vi "camera_config.vi"(7 "Cam Delay":dbl=0.5, 8 "error in (no error)":errorcluster, 9 "Sub Region":T1={"Horizontal Offset"=768, "Vertical Offset"=960, "Horizontal Size"=512, "Vertical Size"=128}, 10 "Exposure Time(s)":dbl=0.00199, 11 "Handle in":u32) -> (0 "error out":errorcluster, 3 "Handle out":u32)   [LabVIEW 2017]
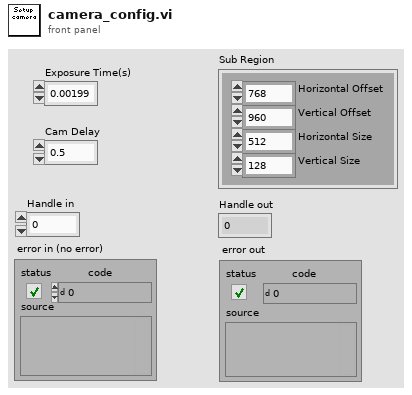
[diagram p1: front panel]
types:
  T1 = cluster{"Horizontal Offset":i32, "Vertical Offset":i32, "Horizontal Size":i32, "Vertical Size":i32}
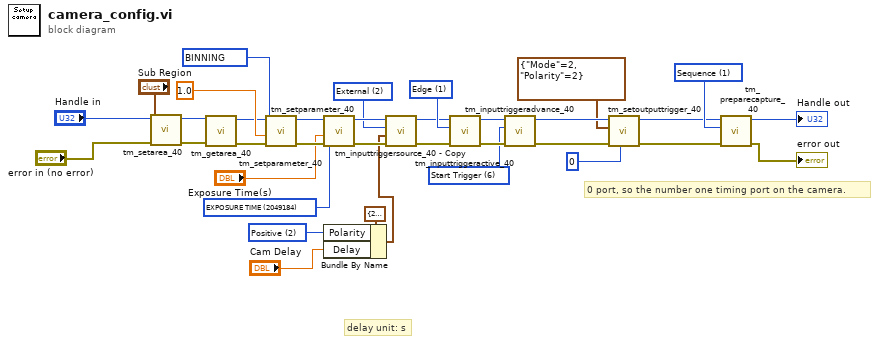
[diagram p0: block diagram]
diagram:
  w3 = 2 items=["Negative"=1, "Positive"=2] ("Polarity")
  w7 = 2 items=["Internal"=1, "External"=2, "Software"=3, "Master Pulse"=4] ("Source")
  w23 = 1 items=["Edge"=1, "Level"=2, "Sync Readout"=3, "Point"=4] ("Active")
  w20 = 6 items=["Normal"=1, "PIV"=3, "Start Trigger"=6, "Multigate"=7, "Multiframe"=8] ("option")
  w24 = 1 items=["Snap", "Sequence"] ("Capture mode")
  w33 = u32 2049184 items=["SENSOR MODE"=4212128, "SENSOR MODE LINE BUNDLE HEIGHT"=4212192, "READOUT DIRECTION"=4211904, "BIT PER CHANNEL"=4342976, "EXPOSURE TIME"=2049184, "CONTRAST GAIN"=3163312, "BINNING"=4215968, "TIMING READOUT TIME"=4223904, "INTERNAL FRAME RATE"=4225952, "INTERNAL FRAME INTERVAL"=4225968, "INTERNAL LINE SPEED"=4226000, "IMAGE WIDTH"=4343200, "IMAGE HEIGHT"=4343216, "IMAGE ROWBYTES"=4343232, "IMAGE FRAMEBYTES"=4343248, "IMAGE PIXEL TYPE"=4343296] ("Parameter")
  w34 = u32 4215968 items=["SENSOR MODE"=4212128, "SENSOR MODE LINE BUNDLE HEIGHT"=4212192, "READOUT DIRECTION"=4211904, "BIT PER CHANNEL"=4342976, "EXPOSURE TIME"=2049184, "CONTRAST GAIN"=3163312, "BINNING"=4215968, "TIMING READOUT TIME"=4223904, "INTERNAL FRAME RATE"=4225952, "INTERNAL FRAME INTERVAL"=4225968, "INTERNAL LINE SPEED"=4226000, "IMAGE WIDTH"=4343200, "IMAGE HEIGHT"=4343216, "IMAGE ROWBYTES"=4343232, "IMAGE FRAMEBYTES"=4343248, "IMAGE PIXEL TYPE"=4343296] ("Parameter")
  # "delay unit: s"
  # "0 port, so the number one timing port on the camera."
  n1 = call <userlib>:"tm_setarea_40.vi"("error in (no error)"="error in (no error)", "Sub Region"="Sub Region", "Handle in"="Handle in") -> ("error out"=w27:errorcluster, "Handle out"=w28:u32)  [unwired: 7 in]
  n2 = call <userlib>:"tm_getarea_40.vi"("error in (no error)"=w27, "Handle in"=w28) -> ("error out"=w25:errorcluster, "Handle out"=w26:u32)  [unwired: 7 in, 1 out]
  n3 = call <userlib>:"tm_setparameter_40.vi"("error in (no error)"=w25, "Value in"=1.0 ("Binning"), "Parameter"=w34, "Handle in"=w26) -> ("error out"=w35:errorcluster, "Handle out"=w29:u32)  [unwired: 6 in]
  n4 = call <userlib>:"tm_setparameter_40.vi"("error in (no error)"=w35, "Value in"="Exposure Time(s)", "Parameter"=w33, "Handle in"=w29) -> ("error out"=w6:errorcluster, "Handle out"=w9:u32)  [unwired: 6 in]
  n5 = Bundle By Name(cluster=cluster{"Polarity":i32, "Delay":dbl} {"Polarity"=2, "Delay"=3.5} ("External Options"), "Polarity"=w3, "Delay"="Cam Delay") -> (w1:cluster{"Polarity":i32, "Delay":dbl})
  n6 = call <userlib>:"tm_inputtriggersource_40 - Copy.vi"("error in (no error)"=w6, "External Options"=w1, "Source"=w7, "Handle in"=w9) -> ("error out"=w5:errorcluster, "Handle out"=w8:u32)  [unwired: 6 in]
  n7 = call <userlib>:"tm_inputtriggeractive_40.vi"("error in (no error)"=w5, "Active"=w23, "Handle in"=w8) -> ("error out"=w21:errorcluster, "Handle out"=w22:u32)  [unwired: 7 in]
  n8 = call <userlib>:"tm_inputtriggeradvance_40.vi"("error in (no error)"=w21, "option"=w20, "Handle in"=w22) -> ("error out"=w13:errorcluster, "Handle out"=w15:u32)  [unwired: 7 in]
  n9 = call <userlib>:"tm_setoutputtrigger_40.vi"("Port"=0, "error in (no error)"=w13, "Type"=cluster{"Mode":u32, "Polarity":u32} {"Mode"=2, "Polarity"=2}, "Handle in"=w15) -> ("error out"=w12:errorcluster, "Handle out"=w14:u32)  [unwired: 6 in]
  n10 = call <userlib>:"tm_preparecapture_40.vi"("error in (no error)"=w12, "Capture mode"=w24, "Handle in"=w14) -> ("error out"=→"error out":errorcluster, "Handle out"=→"Handle out":u32)  [unwired: 5 in, 2 out]
